vi "ACCEL Caculator.vi"(11 "appended array":waveform(dbl)[](array[waveform])) -> (1 "Result":dbl, 2 "Array":dbl[](array[numeric]), 3 "high state level":dbl[](array[numeric]) format="%.2f", 4 "low state level":dbl[](array[numeric]) format="%_6f")   [LabVIEW 2015]
uses:
  <vilib>/measure/mascope.llb/Amplitude and Levels N chan.vi
  <vilib>/express/express arith-compare/Formula/XNode/ExpressFormulaBlockNode.xnode
  <vilib>/measure/NI_MAPro.lvlib
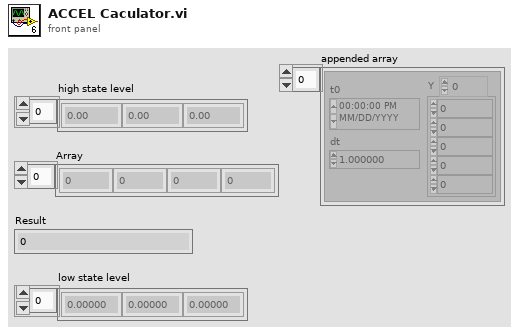
[diagram p1: front panel]
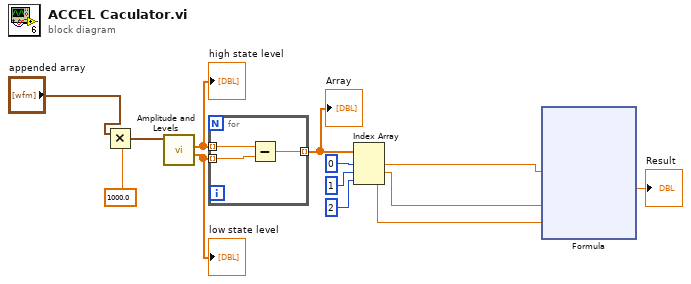
[diagram p0: block diagram]
diagram:
  n1 = Multiply(x="appended array", y=1000.0) -> (x*y=w3:waveform(dbl)[])
  n2 = call-poly <vilib>:"Amplitude and Levels.vi"("signal(s) in"=w3) -> ("low state level"=w5:dbl[], "high state level"=w4:dbl[])  [unwired: 7 in, 2 out]
  "high state level" <- w4
  "low state level" <- w5
  n3 = for {
    tunnel: w4 -> [w16] mode=indexing
    tunnel: w5 -> [w15] mode=indexing
    tunnel: [w14] -> w6 mode=indexing
    n4 = Subtract(x=w16, y=w15) -> (x-y=w14:dbl)
  }
  "Array" <- w6
  n5 = Index Array(array=w6, index #1=0 ("index"), index #2=1 ("index"), index #3=2 ("index")) -> (element #1=w10:dbl, element #2=w11:dbl, element #3=w12:dbl)
  n6 = xnode "Formula"("Xpp"=w10, "Ypp"=w11, "Zpp"=w12) -> ("Result"=→"Result":dbl)  [unwired: 1 in, 1 out]
